vi "PCI1240U初始化.vi"() -> (0 "DevAxesCount":u32, 1 "Y电机":u32, 2 "X电机":u32, 3 "DeviceHandle":u32, 4 "调间隙电机":u32, 5 "进给电机":u32)   [LabVIEW 2013]
panel:
  out "Device Type 2":u16(ring) items=["PCI-1240 (M0)"]
  in  "error in (no error)":errorcluster
  out "error out":errorcluster
  out "AxisOpened":bool
  in  "Device Type":u16(ring) items=["PCI-1220 (M0)"]
  out "DeviceNum List":u32[](array[numeric])
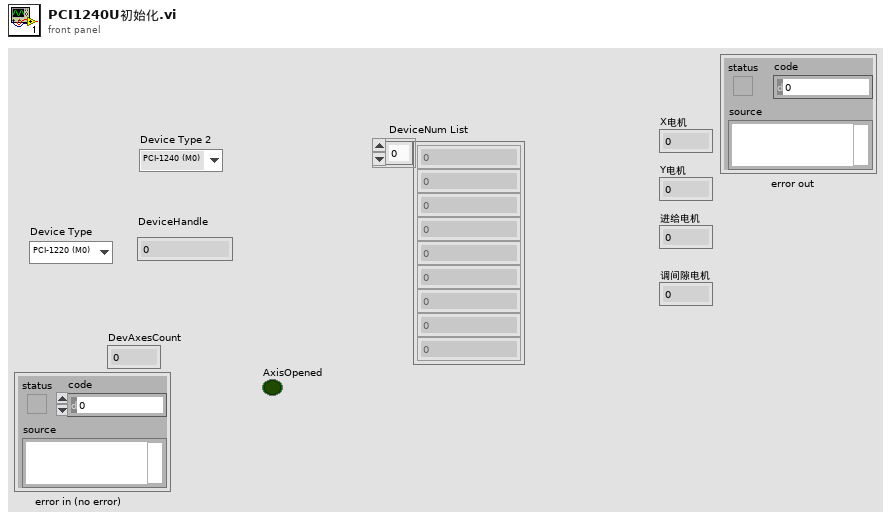
[diagram p1: front panel]
types:
  T1 = cluster{"DeviceNum":u32, "U*8 Array":cluster{"U*8 Array[0]":u8, "U*8 Array[1]":u8, "U*8 Array[2]":u8, "U*8 Array[3]":u8, "U*8 Array[4]":u8, "U*8 Array[5]":u8, "U*8 Array[6]":u8, "U*8 Array[7]":u8, "U*8 Array[8]":u8, "U*8 Array[9]":u8, "U*8 Array[10]":u8, "U*8 Array[11]":u8, "U*8 Array[12]":u8, "U*8 Array[13]":u8, "U*8 Array[14]":u8, "U*8 Array[15]":u8, "U*8 Array[16]":u8, "U*8 Array[17]":u8, "U*8 Array[18]":u8, "U*8 Array[19]":u8, "U*8 Array[20]":u8, "U*8 Array[21]":u8, "U*8 Array[22]":u8, "U*8 Array[23]":u8, "U*8 Array[24]":u8, "U*8 Array[25]":u8, "U*8 Array[26]":u8, "U*8 Array[27]":u8, "U*8 Array[28]":u8, "U*8 Array[29]":u8, "U*8 Array[30]":u8, "U*8 Array[31]":u8, "U*8 Array[32]":u8, "U*8 Array[33]":u8, "U*8 Array[34]":u8, "U*8 Array[35]":u8, "U*8 Array[36]":u8, "U*8 Array[37]":u8, "U*8 Array[38]":u8, "U*8 Array[39]":u8, "U*8 Array[40]":u8, "U*8 Array[41]":u8, "U*8 Array[42]":u8, "U*8 Array[43]":u8, "U*8 Array[44]":u8, "U*8 Array[45]":u8, "U*8 Array[46]":u8, "U*8 Array[47]":u8, "U*8 Array[48]":u8, "U*8 Array[49]":u8}, "NumOfSubDevice":i16}[]
  T2 = cluster{"U*8 Array[0]":u8, "U*8 Array[1]":u8, "U*8 Array[2]":u8, "U*8 Array[3]":u8, "U*8 Array[4]":u8, "U*8 Array[5]":u8, "U*8 Array[6]":u8, "U*8 Array[7]":u8, "U*8 Array[8]":u8, "U*8 Array[9]":u8, "U*8 Array[10]":u8, "U*8 Array[11]":u8, "U*8 Array[12]":u8, "U*8 Array[13]":u8, "U*8 Array[14]":u8, "U*8 Array[15]":u8, "U*8 Array[16]":u8, "U*8 Array[17]":u8, "U*8 Array[18]":u8, "U*8 Array[19]":u8, "U*8 Array[20]":u8, "U*8 Array[21]":u8, "U*8 Array[22]":u8, "U*8 Array[23]":u8, "U*8 Array[24]":u8, "U*8 Array[25]":u8, "U*8 Array[26]":u8, "U*8 Array[27]":u8, "U*8 Array[28]":u8, "U*8 Array[29]":u8, "U*8 Array[30]":u8, "U*8 Array[31]":u8, "U*8 Array[32]":u8, "U*8 Array[33]":u8, "U*8 Array[34]":u8, "U*8 Array[35]":u8, "U*8 Array[36]":u8, "U*8 Array[37]":u8, "U*8 Array[38]":u8, "U*8 Array[39]":u8, "U*8 Array[40]":u8, "U*8 Array[41]":u8, "U*8 Array[42]":u8, "U*8 Array[43]":u8, "U*8 Array[44]":u8, "U*8 Array[45]":u8, "U*8 Array[46]":u8, "U*8 Array[47]":u8, "U*8 Array[48]":u8, "U*8 Array[49]":u8}
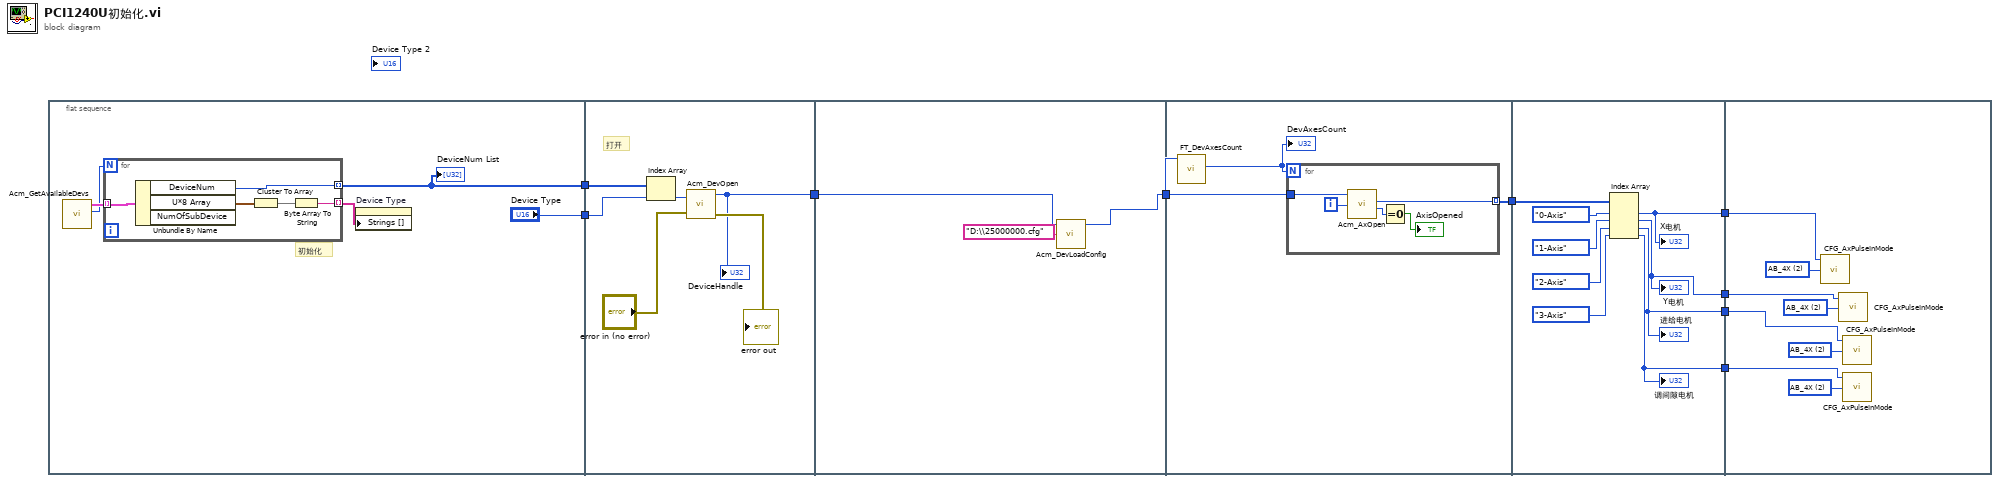
[diagram p0: block diagram]
diagram:
  n1 = flat-sequence {
    tunnel: [w13] -> w9
    tunnel: ["Device Type"] -> w8
    tunnel: w9 -> [w25]
    tunnel: w8 -> [w23]
    tunnel: [w20] -> w2
    tunnel: w2 -> [w28]
    tunnel: [w26] -> w1
    tunnel: w1 -> [w30]
    tunnel: [w29] -> w7
    tunnel: w7 -> [w45]
    tunnel: [w43] -> w6
    tunnel: [w39] -> w5
    tunnel: [w38] -> w4
    tunnel: [w37] -> w3
    tunnel: w6 -> [w46]
    tunnel: w5 -> [w49]
    tunnel: w4 -> [w48]
    tunnel: w3 -> [w47]
    frame #0 {
      # "初始化"
      n2 = call <userlib>:"Acm_GetAvailableDevs.vi"() -> ("OutEntries"=w10:u32, "DeviceList"=w11:T1)  [unwired: 1 in, 2 out]
      n3 = for {
        N: w10 -> [_]
        tunnel: w11 -> [w19] mode=indexing
        tunnel: [w16] -> w13 mode=indexing
        tunnel: [w15] -> w14 mode=indexing
        n4 = Unbundle By Name(w19) -> ("DeviceNum"=w16:u32, "U*8 Array"=w18:T2)  [unwired: 1 out]
        n5 = Cluster To Array(cluster=w18) -> (array=w17:u8[])
        n6 = Byte Array To String(unsigned byte array=w17) -> (string=w15:string)
      }
      "DeviceNum List" <- w13
      n7 = property on="Device Type" class="Ring (严格)"("Strings []"=w14) -> ()  [unwired: 2 in, 2 out]
    }
    frame #1 {
      # "打开"
      n8 = Index Array(array=w25, index=w23) -> (element=w24:u32)
      n9 = call <userlib>:"Acm_DevOpen.vi"("Error Input(No Error)"="error in (no error)", "DeviceNumber"=w24) -> ("Error Output"=→"error out":errorcluster, "DeviceHandle"=w20:u32)  [unwired: 1 out]
      "DeviceHandle" <- w20
    }
    frame #2 {
      n10 = call <userlib>:"Acm_DevLoadConfig.vi"("ConfigPath"="D:\\25000000.cfg", "DeviceHandle"=w28) -> ("DeviceHandle"=w26:u32)  [unwired: 1 in, 2 out]
    }
    frame #3 {
      n11 = call <userlib>:"FT_DevAxesCount.vi"("Handle"=w30) -> ("DevAxesCount"=w31:u32)  [unwired: 3 in, 4 out]
      "DevAxesCount" <- w31
      n12 = for {
        N: w31 -> [_]
        tunnel: w30 -> [w36]
        tunnel: [w32] -> w29 mode=indexing
        i -> [w35]
        n13 = call <userlib>:"Acm_AxOpen.vi"("PhyAxis"=w35, "DeviceHandle"=w36) -> ("ReturnValue"=w34:u32, "AxisHandle"=w32:u32)  [unwired: 1 in, 2 out]
        n14 = Equal To 0?(x=w34) -> (x = 0?=→"AxisOpened":bool)
      }
    }
    frame #4 {
      n15 = Index Array(array=w45, index #1=enum32{"0-Axis", "1-Axis", "2-Axis", "3-Axis"}."0-Axis" ("Operate Axis"), index #2=enum32{"0-Axis", "1-Axis", "2-Axis", "3-Axis"}."1-Axis" ("Operate Axis"), index #3=enum32{"0-Axis", "1-Axis", "2-Axis", "3-Axis"}."2-Axis" ("Operate Axis"), index #4=enum32{"0-Axis", "1-Axis", "2-Axis", "3-Axis"}."3-Axis" ("Operate Axis")) -> (element #1=w43:u32, element #2=w39:u32, element #3=w38:u32, element #4=w37:u32)
      "X电机" <- w43
      "Y电机" <- w39
      "进给电机" <- w38
      "调间隙电机" <- w37
    }
    frame #5 {
      w50 = u32 2 items=["AB_1X", "AB_2X", "AB_4X", "I_CW_CCW"] ("CFG_AxPulseInMode")
      w51 = u32 2 items=["AB_1X", "AB_2X", "AB_4X", "I_CW_CCW"] ("CFG_AxPulseInMode")
      w52 = u32 2 items=["AB_1X", "AB_2X", "AB_4X", "I_CW_CCW"] ("CFG_AxPulseInMode")
      w53 = u32 2 items=["AB_1X", "AB_2X", "AB_4X", "I_CW_CCW"] ("CFG_AxPulseInMode")
      n16 = call <userlib>:"CFG_AxPulseInMode.vi"("CFG_AxPulseInMode"=w53, "Handle"=w46) -> ()  [unwired: 1 in, 3 out]
      n17 = call <userlib>:"CFG_AxPulseInMode.vi"("CFG_AxPulseInMode"=w52, "Handle"=w49) -> ()  [unwired: 1 in, 3 out]
      n18 = call <userlib>:"CFG_AxPulseInMode.vi"("CFG_AxPulseInMode"=w51, "Handle"=w48) -> ()  [unwired: 1 in, 3 out]
      n19 = call <userlib>:"CFG_AxPulseInMode.vi"("CFG_AxPulseInMode"=w50, "Handle"=w47) -> ()  [unwired: 1 in, 3 out]
    }
  }
